vi "Check for All Content.vi"(8 "error in (no error)":errorcluster, 11 "data in":string="POST / HTTP/1.0\r\nContent-Type: text/xml\r\nUser-Agent: XML-RPC.NET\r\nHost: s881643.srn.sandia.gov:8080\r\nContent-Length: 212\r\nVia: 1.1 sahp4060.sandia.gov:80 (squid/2.5.STABLE9)\r\nX-Forwarded-For: 134.253.202.68\r\nCache-Control: max-age=259200\r\nConnection: keep-alive\r\n\r\n<?xml version=\"1.0\"?>\r\n<methodCall>\r\n  <methodName>Dialog Test.vi</methodName>\r\n  <params>\r\n    <param>\r\n      <value>\r\n        <string>asdasdsad</string>\r\n      </value>\r\n    </param>\r\n  </params>\r\n</methodCall>\r\n") -> (0 "error out":errorcluster, 3 "all content read":bool)   [LabVIEW 2014]
doc: "This VI checks the data actually read against the Content-Length specified and returns an error if less bytes than specified in Content-Length are read"
panel:
  out "Content-Length":i32
  out "length":i32
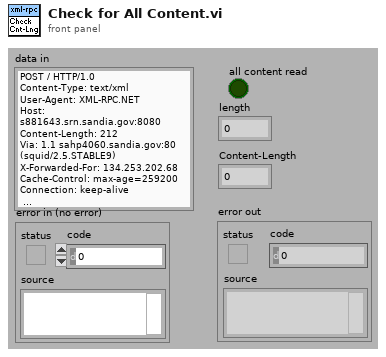
[diagram p1: front panel]
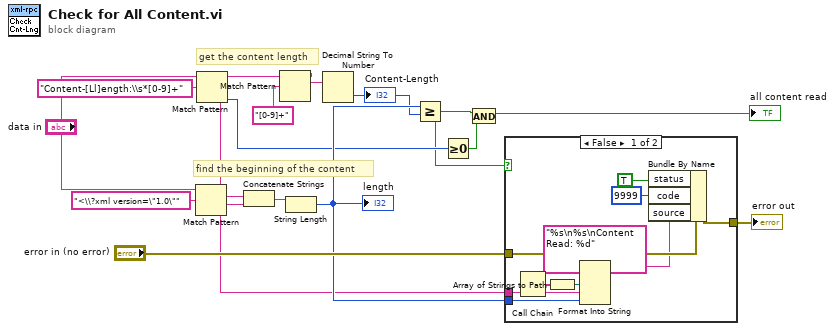
[diagram p0: block diagram]
diagram:
  # "find the beginning of the content"
  # "get the content length"
  n1 = Match Pattern(string="data in", regular expression="<\\?xml version=\"1.0\"") -> (match substring=w12:string, after substring=w11:string)  [unwired: 1 in, 2 out]
  n2 = Match Pattern(string="data in", regular expression="Content-[Ll]ength:\\s*[0-9]+") -> (match substring=w6:string, offset past match=w4:i32)  [unwired: 1 in, 2 out]
  n3 = Concatenate Strings(w12, w11) -> (w10:string)
  n4 = Match Pattern(string=w6, regular expression="[0-9]+") -> (match substring=w15:string)  [unwired: 1 in, 3 out]
  n5 = String Length(string=w10) -> (length=w7:i32)
  "length" <- w7
  n6 = Decimal String To Number(string=w15) -> (number=w5:i32)  [unwired: 2 in, 1 out]
  "Content-Length" <- w5
  n7 = Greater Or Equal?(x=w7, y=w5) -> (x >= y?=w3:bool)
  n8 = Greater Or Equal To 0?(x=w4) -> (x >= 0?=w2:bool)
  n9 = And(x=w3, y=w2) -> (x .and. y?=→"all content read":bool)
  n10 = case shown="False" w3 {
    tunnel: "error in (no error)" -> [w26 w28]
    tunnel: [w22 w28] -> w8
    tunnel: w6 -> [w19 _]
    tunnel: w7 -> [w18 _]
    frame False {
      n11 = Call Chain() -> (call chain=w27:string[])
      n12 = Array of Strings to Path(0:w27) -> (2:w23:path)  [unwired: 1 in]
      n13 = Format Into String(format string="%s\n%s\nContent Read: %d", w23, w19, w18) -> (resulting string=w21:string)  [unwired: 2 in, 1 out]
      n14 = Bundle By Name(cluster=w26, "status"=TRUE, "code"=9999, "source"=w21) -> (w22:errorcluster)
    }
    frame True {
    }
  }
  "error out" <- w8
